vi "2-12.vi"() -> ()   [LabVIEW 2022 SP3]
panel:
  out "数值":dbl
  out "字符串":string
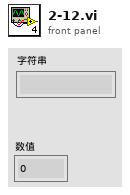
[diagram p1: front panel]
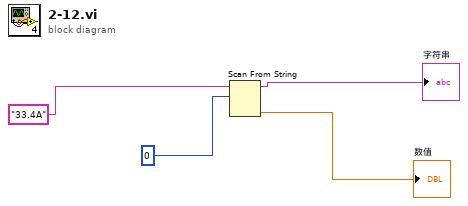
[diagram p0: block diagram]
diagram:
  n1 = Scan From String(input string="33.4A", initial scan location=0) -> (remaining string=→"字符串":string, output 1=→"数值":dbl)  [unwired: 3 in, 2 out]
